vi "AutomatedTestTemplate.vi"() -> ()   [LabVIEW 2014]
uses:
  Utilities/ControlValues/ControlValues.lvclass
  Controls/Config.ctl
  Utilities/DataShare/DataShare.lvclass
  <vilib>/Utility/error.llb/DialogType.ctl
  Controls/Data.ctl
panel:
  in  "SelectPanel":i32(listbox)=-1
  out "Data":string[][](table)
  out "Status":string
  # "Blank area for constantly available displays"
  # "Blank area for constantly available displays, delete splitter if not needed"
  # "Blank area for constantly available displays"
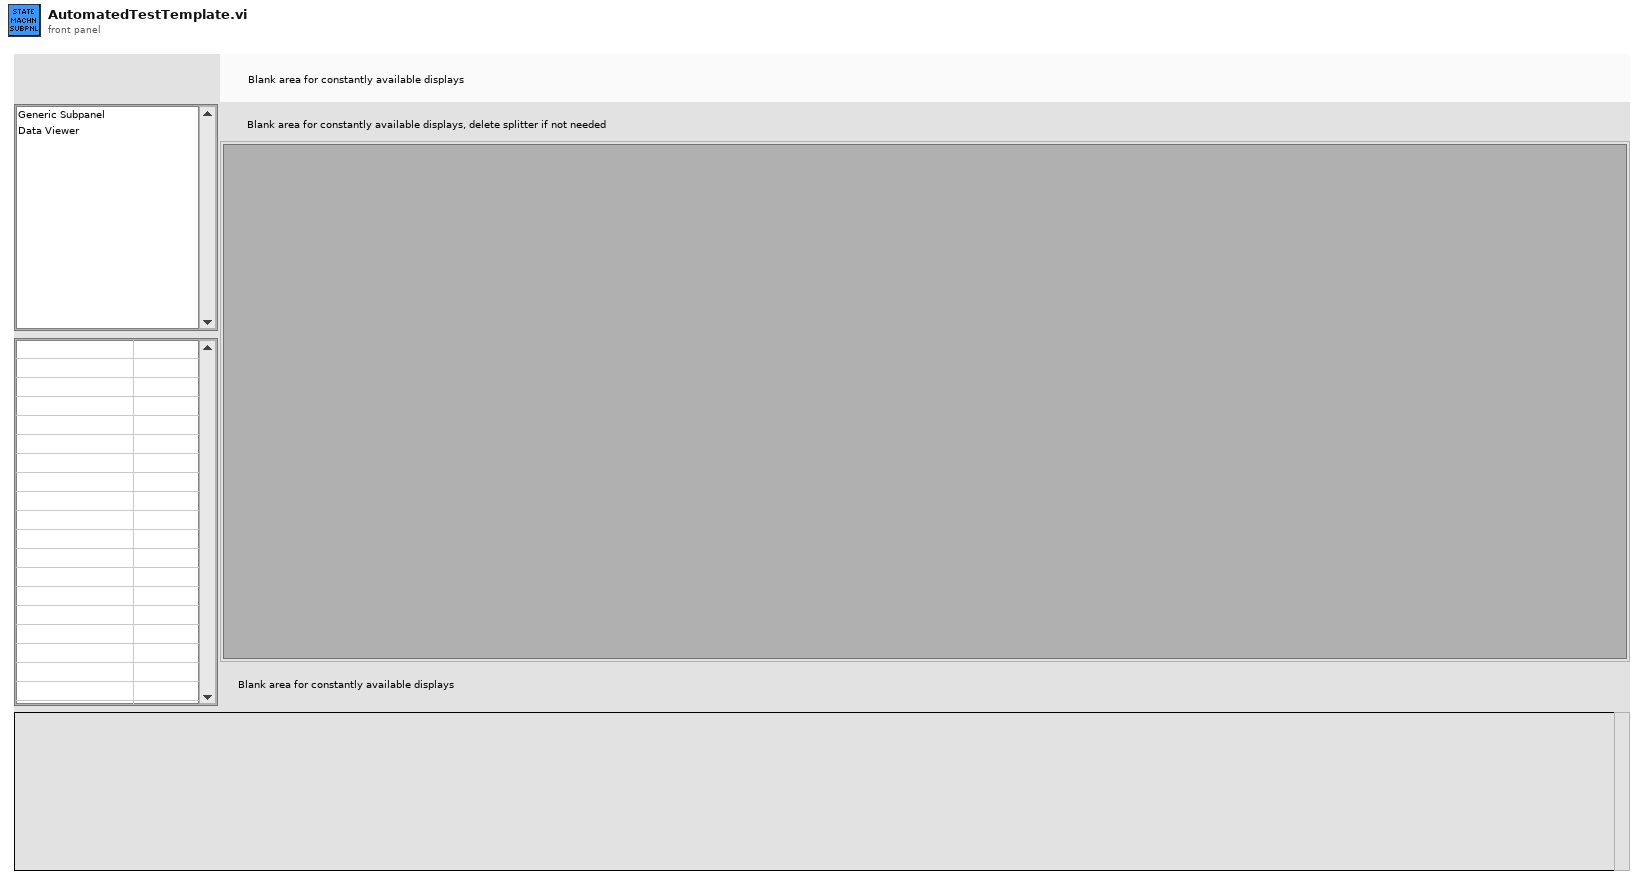
[diagram p1: front panel]
types:
  T1 = typedef "Config.ctl" = cluster{"Subpanels":cluster{"Name":string, "Pathname":string, "Type":string}[]}
  T2 = cluster{"Error":errorcluster, "SubpanelRefs":refnum<vi>[], "SubpanelRef":refnum<vi>, "ControlValues":refnum<class "ControlValues.lvclass">, "AppKind":enum32{"invalid app kind", "Development System", "Run Time System", "Student Edition", "Embedded LabVIEW", "Evaluation", "Custom"}, "LogFolder":path, "ConfigFolder":path, "Config":T1, "Hidden":T1, "Visible":T1, "Example":refnum<class "DataShare.lvclass">}
  T3 = typedef "Data.ctl" = cluster{"Names":string[], "Values":dbl[]}
  T4 = enum32{"invalid app kind", "Development System", "Run Time System", "Student Edition", "Embedded LabVIEW", "Evaluation", "Custom"}
  T5 = cluster{"Name":string, "Pathname":string, "Type":string}[]
  T6 = typedef "DialogType.ctl" = u16
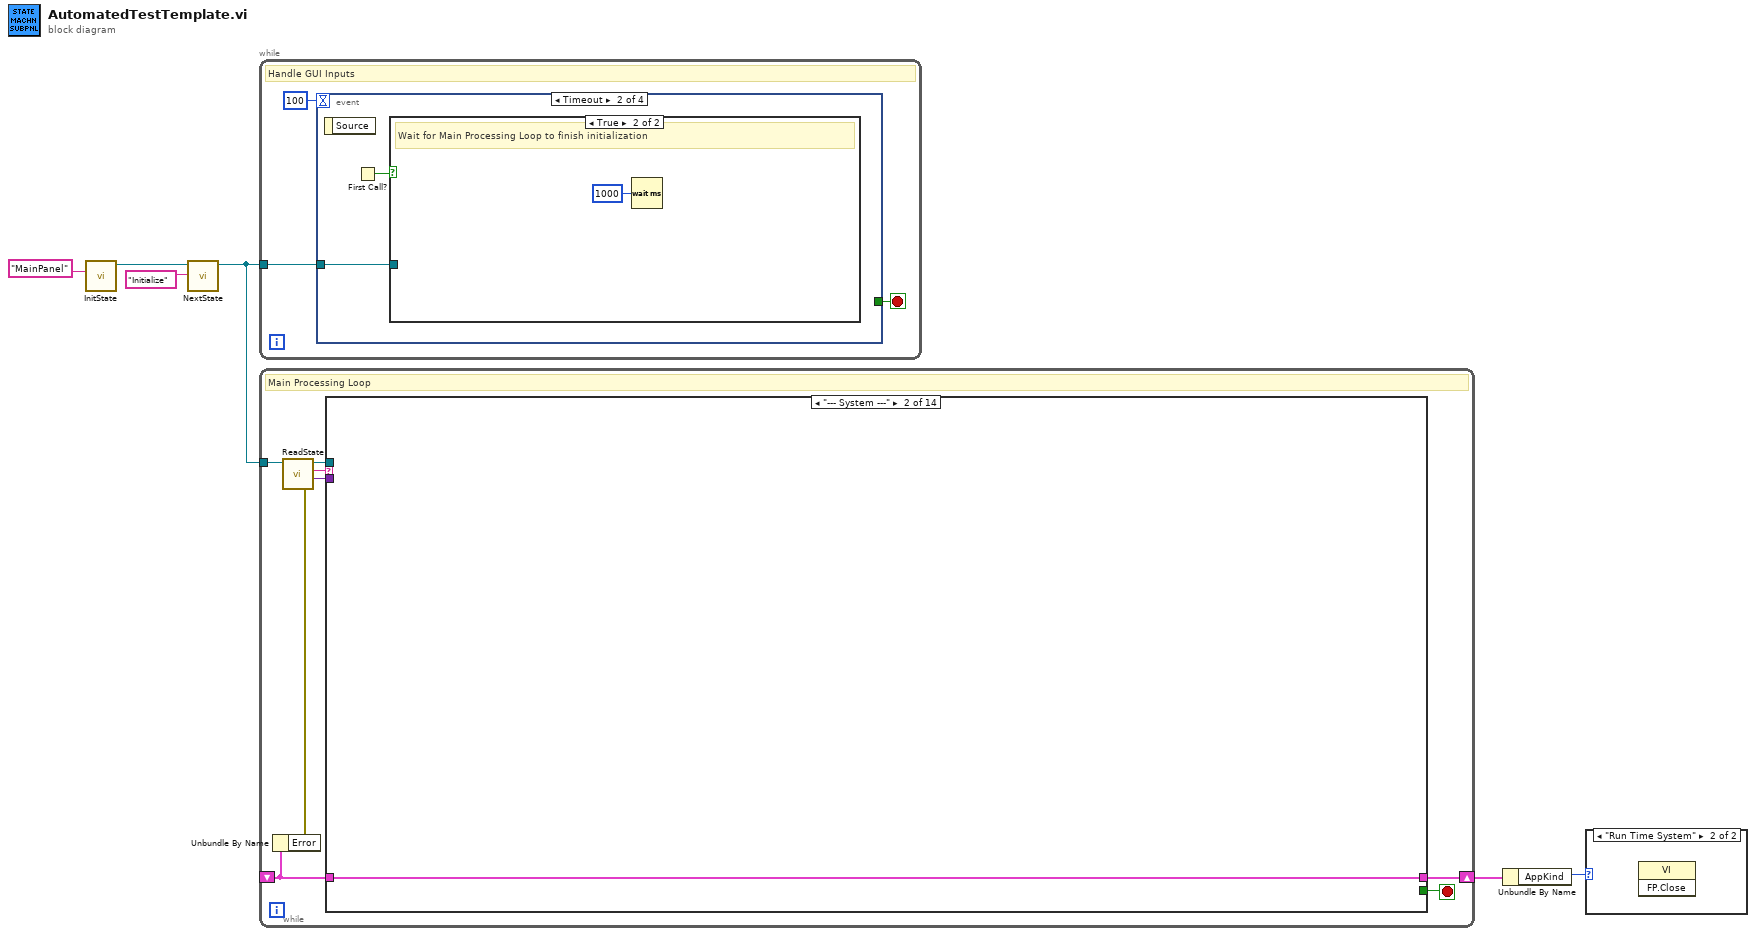
[diagram p0: block diagram]
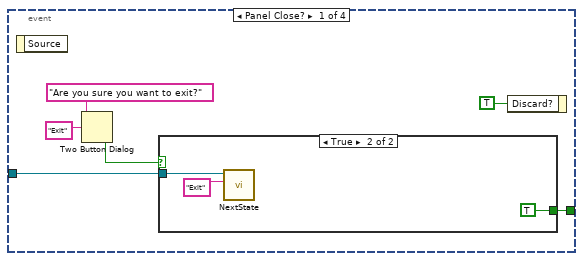
[diagram p3: hidden frame]
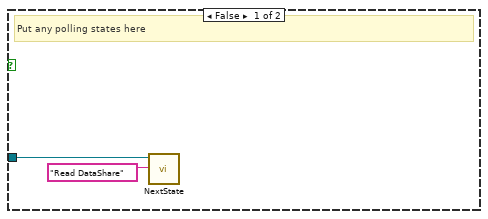
[diagram p5: hidden frame]
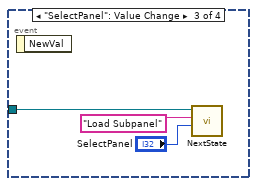
[diagram p6: hidden frame]
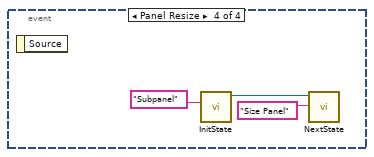
[diagram p7: hidden frame]
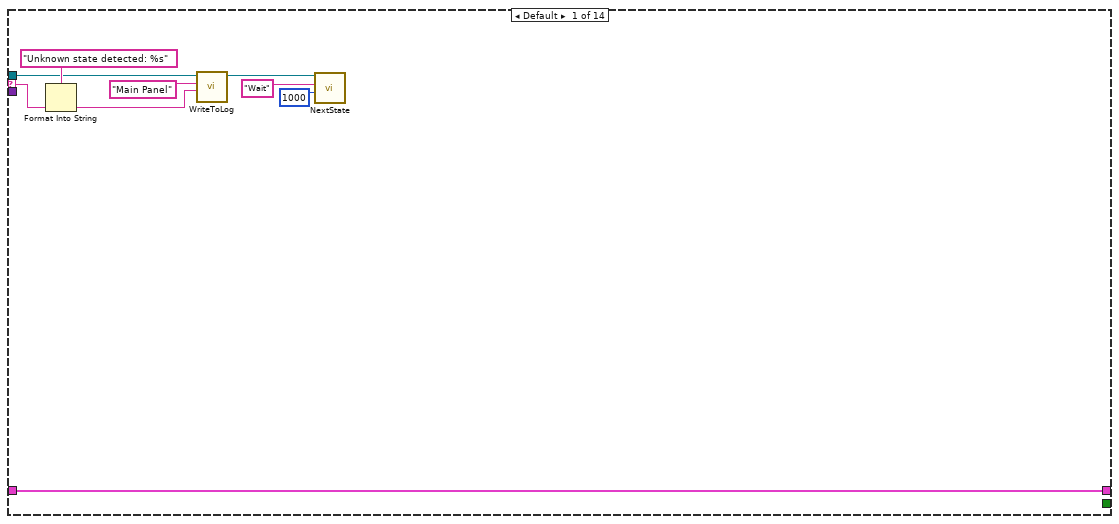
[diagram p8: hidden frame]
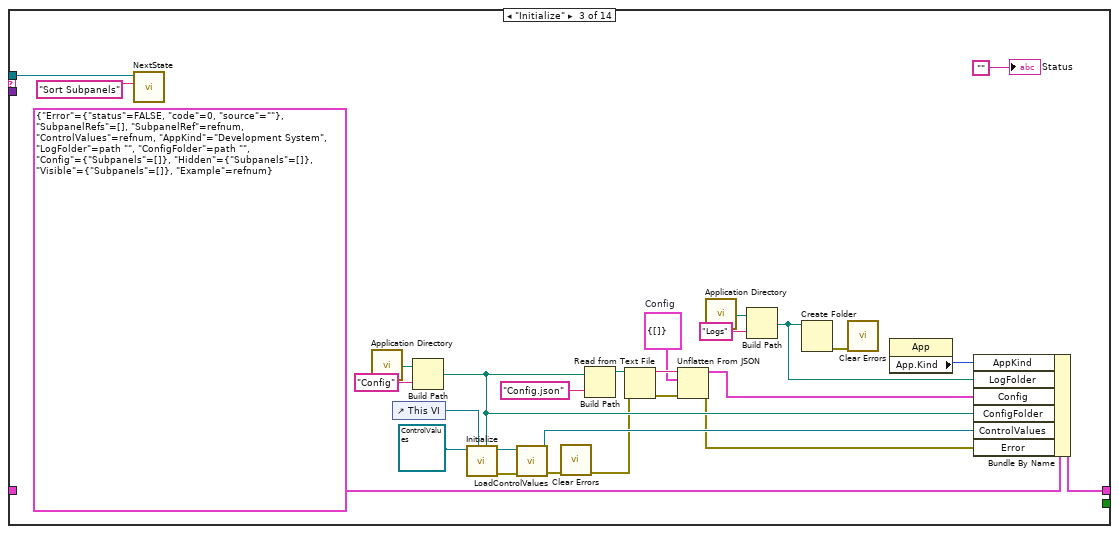
[diagram p9: hidden frame]
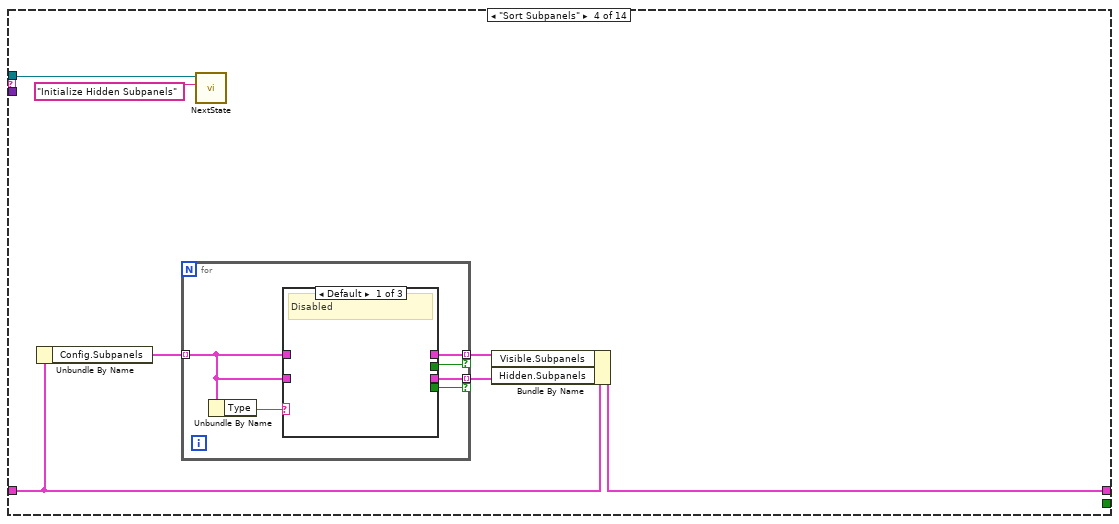
[diagram p10: hidden frame]
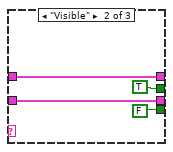
[diagram p11: hidden frame]
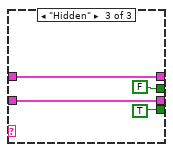
[diagram p12: hidden frame]
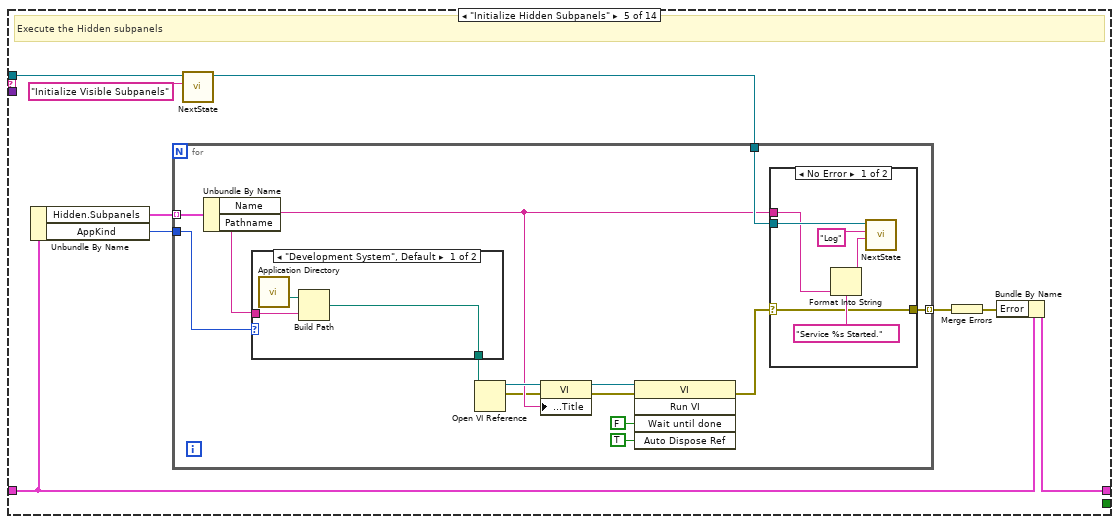
[diagram p13: hidden frame]
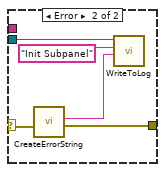
[diagram p14: hidden frame]
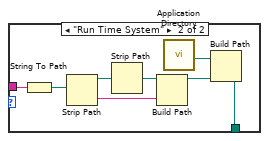
[diagram p15: hidden frame]
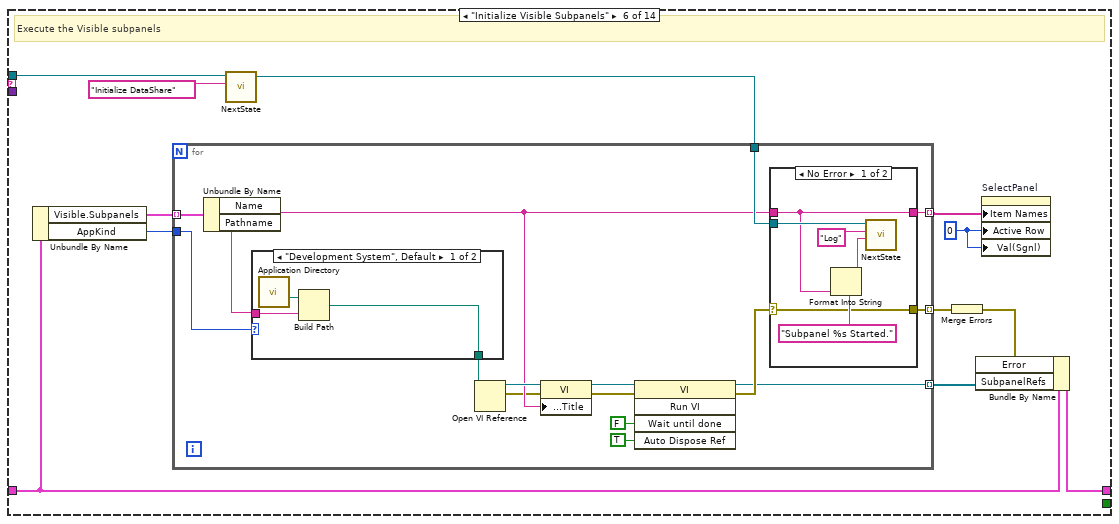
[diagram p16: hidden frame]
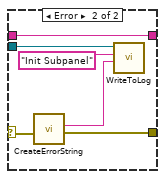
[diagram p17: hidden frame]
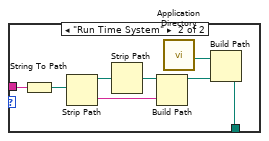
[diagram p18: hidden frame]
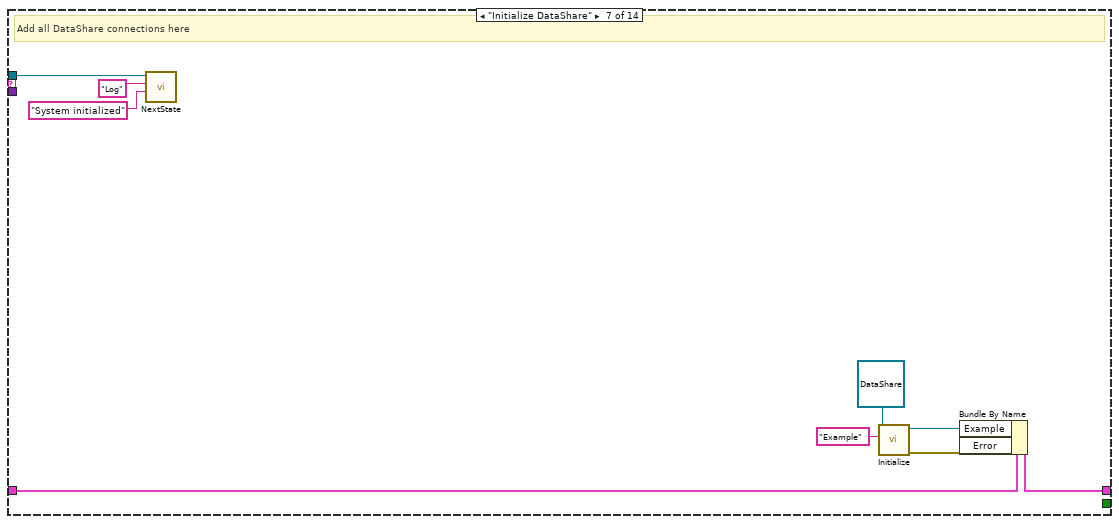
[diagram p19: hidden frame]
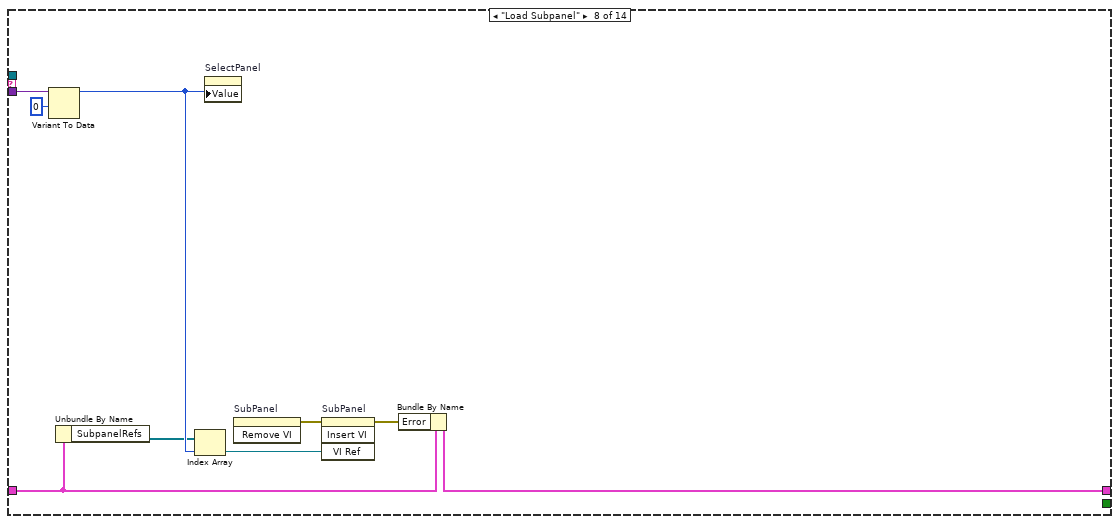
[diagram p20: hidden frame]
diagram:
  n1 = call "InitState.vi"("Name"="MainPanel" ("name (unnamed)")) -> ("Queue Out"=w2:refnum<queue>)  [unwired: 8 in, 1 out]
  n2 = call "NextState.vi"("State"="Initialize" ("element"), "Queue In"=w2) -> ("Queue Out"=w1:refnum<queue>)  [unwired: 8 in, 1 out]
  n3 = while {
    tunnel: w1 -> [w9]
    stop <- w8 stop-if-true
    # "Handle GUI Inputs"
    n4 = event shown="[1] Timeout" {
      selector: _ -> [_ _ _ _]
      dyn-events: _ -> [_ _ _ _]
      timeout: 100 -> [_ _ _ _]
      tunnel: w9 -> [w15 w19 w25 _]
      tunnel: [w10 _ _ _] -> w8
      event Panel Close? {
        n5 = event-data() -> ()  [unwired: 1 in, 1 out]
        n6 = Two Button Dialog(message="Are you sure you want to exit?", 2:"Exit" ("T button name (\"OK\")")) -> (T button?=w11:bool)  [unwired: 1 in]
        n7 = case shown="True" w11 {
          tunnel: w15 -> [_ w16]
          tunnel: [_ TRUE] -> w10
          frame False {
          }
          frame True {
            n8 = call "NextState.vi"("State"="Exit" ("element"), "Queue In"=w16) -> ()  [unwired: 8 in, 2 out]
          }
        }
        n9 = event-data("Discard?"=TRUE) -> ()  [unwired: 1 in, 1 out]
      }
      event Timeout {
        n10 = event-data() -> ()  [unwired: 1 in, 1 out]
        n11 = First Call?() -> (First Call?: T/F=w20:bool)
        n12 = case shown="True" w20 {
          tunnel: w19 -> [w22 _]
          frame False {
            # "Put any polling states here"
            n13 = call "NextState.vi"("State"="Read DataShare" ("element"), "Queue In"=w22) -> ()  [unwired: 8 in, 2 out]
          }
          frame True {
            # "Wait for Main Processing Loop to finish initialization"
            n14 = Wait (ms)(milliseconds to wait=u32 1000) -> ()  [unwired: 1 out]
          }
        }
      }
      event "SelectPanel": Value Change {
        n15 = event-data() -> ()  [unwired: 1 in, 1 out]
        n16 = call "NextState.vi"("Data"="SelectPanel", "State"="Load Subpanel", "Queue In"=w25) -> ()  [unwired: 7 in, 2 out]
      }
      event Panel Resize {
        n17 = event-data() -> ()  [unwired: 1 in, 1 out]
        n18 = call "InitState.vi"("Name"="Subpanel" ("name (unnamed)")) -> ("Queue Out"=w27:refnum<queue>)  [unwired: 8 in, 1 out]
        n19 = call "NextState.vi"("State"="Size Panel" ("element"), "Queue In"=w27) -> ()  [unwired: 8 in, 2 out]
      }
    }
  }
  n20 = while {
    tunnel: w1 -> [w35]
    shift-right: [w37] -> w6
    shift-left: _ -> [w31]
    stop <- w36 stop-if-true
    # "Main Processing Loop"
    n21 = Unbundle By Name(w31) -> ("Error"=w30:errorcluster)
    n22 = call "ReadState.vi"("Error In"=w30, "Queue In"=w35) -> ("Data"=w32:variant, "State"=w33:string, "Queue Out"=w34:refnum<queue>)  [unwired: 6 in, 1 out]
    n23 = case shown="\"--- System ---\"" w33 {
      tunnel: w34 -> [w43 _ w49 w76 w98 w142 w192 _ _ _ w258 w278 _ _]
      tunnel: w32 -> [_ _ _ _ _ _ _ w208 w224 w237 w245 _ _ _]
      selector: w33 -> [w45 _ _ _ _ _ _ _ _ _ _ _ _ _]
      tunnel: [w44 w47 w74 w77 w101 w146 w196 w206 w213 w234 w260 w277 w290 w295] -> w37
      tunnel: [_ _ _ _ _ _ _ _ _ _ _ TRUE _ _] -> w36
      tunnel: w31 -> [w44 w47 _ w80 w102 w147 w197 w205 w213 w234 w241 w277 w290 w295]
      frame Default {
        n24 = Format Into String(format string="Unknown state detected: %s", w45) -> (resulting string=w38:string)  [unwired: 2 in, 1 out]
        n25 = call "WriteToLog.vi"("Data"=w38, "Source"="Main Panel", "Queue In"=w43) -> ("Queue Out"=w42:refnum<queue>)  [unwired: 7 in, 1 out]
        n26 = call "NextState.vi"("Data"=u32 1000, "State"="Wait", "Queue In"=w42) -> ()  [unwired: 7 in, 2 out]
      }
      frame "--- System ---" {
      }
      frame "Initialize" {
        w53 = T1 {"Subpanels"=[]}  # Config
        n27 = call "NextState.vi"("State"="Sort Subpanels" ("element"), "Queue In"=w49) -> ()  [unwired: 8 in, 2 out]
        n28 = call <vilib>:"Application Directory.vi"() -> ("Application Directory"=w62:path)
        n29 = control-ref of="This VI"() -> (w69:refnum<vi>)
        n30 = Build Path(base path=w62, name or relative path="Config") -> (appended path=w57:path)
        n31 = call "Initialize.vi"("Config Path"=w57, "VI Reference"=w69, "ControlValues in"=refnum<class "ControlValues.lvclass"> refnum) -> ("error out"=w71:errorcluster, "ControlValues out"=w72:refnum<class "ControlValues.lvclass">)  [unwired: 7 in]
        n32 = call "LoadControlValues.vi"("error in"=w71, "ControlValues in"=w72) -> ("error out"=w64:errorcluster, "ControlValues out"=w70:refnum<class "ControlValues.lvclass">)  [unwired: 8 in]
        n33 = call <vilib>:"Clear Errors.vi"("error in (no error)"=w64) -> ("error out"=w54:errorcluster)  [unwired: 5 in, 1 out]
        n34 = Build Path(base path=w57, name or relative path="Config.json") -> (appended path=w58:path)
        n35 = Read from Text File(file (use dialog)=w58, error in=w54) -> (text=w59:string, error out=w60:errorcluster)  [unwired: 2 in, 2 out]
        n36 = Unflatten From JSON(JSON string=w59, type and defaults=w53, error in (no error)=w60) -> (value=w52:T1, error out=w50:errorcluster)  [unwired: 4 in]
        n37 = call <vilib>:"Application Directory.vi"() -> ("Application Directory"=w67:path)
        n38 = Build Path(base path=w67, name or relative path="Logs") -> (appended path=w56:path)
        n39 = Create Folder(path (use dialog)=w56) -> (error out=w65:errorcluster)  [unwired: 2 in, 2 out]
        n40 = call <vilib>:"Clear Errors.vi"("error in (no error)"=w65) -> ()  [unwired: 5 in, 2 out]
        n41 = property class="App"() -> ("App.Kind"=w51:T4)  [unwired: 2 in, 2 out]
        n42 = Bundle By Name(cluster=T2 {"Error"={"status"=FALSE, "code"=0, "source"=""}, "SubpanelRefs"=[], "SubpanelRef"=refnum, "ControlValues"=refnum, "AppKind"=enum."Development System", "LogFolder"=path "", "ConfigFolder"=path "", "Config"={"Subpanels"=[]}, "Hidden"={"Subpanels"=[]}, "Visible"={"Subpanels"=[]}, "Example"=refnum}, "AppKind"=w51, "LogFolder"=w56, "Config"=w52, "ConfigFolder"=w57, "ControlValues"=w70, "Error"=w50) -> (w74:T2)
        "Status" <- ""
      }
      frame "Sort Subpanels" {
        n43 = Unbundle By Name(w80) -> ("Config.Subpanels"=w81:T5)
        n44 = for {
          tunnel: w81 -> [w86] mode=indexing
          tunnel: [w85] -> w79 mode=indexing if=w82
          tunnel: [w84] -> w78 mode=indexing if=w83
          n45 = Unbundle By Name(w86) -> ("Type"=w87:string)
          n46 = case shown="Default" w87 {
            tunnel: [_ w91 w95] -> w85
            tunnel: w86 -> [_ w91 w95]
            tunnel: w86 -> [_ w90 w94]
            tunnel: [_ w90 w94] -> w84
            tunnel: [_ TRUE FALSE] -> w82
            tunnel: [_ FALSE TRUE] -> w83
            frame Default {
              # "Disabled"
            }
            frame "Visible" {
            }
            frame "Hidden" {
            }
          }
        }
        n47 = call "NextState.vi"("State"="Initialize Hidden Subpanels" ("element"), "Queue In"=w76) -> ()  [unwired: 8 in, 2 out]
        n48 = Bundle By Name(cluster=w80, "Visible.Subpanels"=w79, "Hidden.Subpanels"=w78) -> (w77:T2)
      }
      frame "Initialize Hidden Subpanels" {
        # "Execute the Hidden subpanels"
        n49 = Unbundle By Name(w102) -> ("Hidden.Subpanels"=w104:T5, "AppKind"=w103:T4)
        n50 = call "NextState.vi"("State"="Initialize Visible Subpanels", "Queue In"=w98) -> ("Queue Out"=w97:refnum<queue>)  [unwired: 8 in, 1 out]
        n51 = for {
          tunnel: w104 -> [w118] mode=indexing
          tunnel: w103 -> [w116]
          tunnel: w97 -> [w115]
          tunnel: [w105] -> w100 mode=indexing
          n52 = Unbundle By Name(w118) -> ("Name"=w109:string, "Pathname"=w117:string)
          n53 = case shown="\"Development System\", Default" w116 {
            tunnel: w117 -> [w131 w140]
            tunnel: [w130 w134] -> w114
            frame "Development System", Default {
              n54 = call <vilib>:"Application Directory.vi"() -> ("Application Directory"=w132:path)
              n55 = Build Path(base path=w132, name or relative path=w131) -> (appended path=w130:path)
            }
            frame "Run Time System" {
              n56 = String To Path(string=w140) -> (path=w139:path)
              n57 = Strip Path(path=w139) -> (stripped path=w138:path, name=w137:string)
              n58 = Strip Path(path=w138) -> (stripped path=w136:path)  [unwired: 1 out]
              n59 = Build Path(base path=w136, name or relative path=w137) -> (appended path=w135:path)
              n60 = call <vilib>:"Application Directory.vi"() -> ("Application Directory"=w133:path)
              n61 = Build Path(base path=w133, name or relative path=w135) -> (appended path=w134:path)
            }
          }
          n62 = Open VI Reference(vi path=w114) -> (vi reference=w110:refnum<vi>, error out=w106:errorcluster)  [unwired: 5 in]
          n63 = property class="VI"(reference=w110, error in=w106, "Front Panel.Title"=w109) -> (reference out=w108:refnum<vi>, error out=w107:errorcluster)
          n64 = invoke class="VI" method="Run VI"(reference=w108, error in=w107, "Wait until done"=FALSE ("Wait Until Done"), "Auto Dispose Ref"=TRUE ("Auto Dispose Reference")) -> (error out=w111:errorcluster)  [unwired: 1 in, 4 out]
          n65 = case shown="No Error" w111 {
            selector: w111 -> [w119 w129]
            tunnel: w115 -> [w123 w128]
            tunnel: w109 -> [w120 _]
            tunnel: [w119 w125] -> w105
            frame No Error {
              n66 = Format Into String(format string="Service %s Started.", w120) -> (resulting string=w121:string)  [unwired: 2 in, 1 out]
              n67 = call "NextState.vi"("Data"=w121, "State"="Log" ("element"), "Queue In"=w123) -> ()  [unwired: 7 in, 2 out]
            }
            frame Error {
              n68 = call "CreateErrorString.vi"("Error In"=w129) -> ("Error Out"=w125:errorcluster, "Error String"=w126:string)  [unwired: 9 in]
              n69 = call "WriteToLog.vi"("Data"=w126, "Source"="Init Subpanel", "Queue In"=w128) -> ()  [unwired: 7 in, 2 out]
            }
          }
        }
        n70 = Merge Errors(w100) -> (w99:errorcluster)
        n71 = Bundle By Name(cluster=w102, "Error"=w99) -> (w101:T2)
      }
      frame "Initialize Visible Subpanels" {
        w150 = 0 ("Active Row:Active Row Number")
        # "Execute the Visible subpanels"
        n72 = Unbundle By Name(w147) -> ("Visible.Subpanels"=w152:T5, "AppKind"=w151:T4)
        n73 = call "NextState.vi"("State"="Initialize DataShare" ("element"), "Queue In"=w142) -> ("Queue Out"=w141:refnum<queue>)  [unwired: 8 in, 1 out]
        n74 = for {
          tunnel: w152 -> [w168] mode=indexing
          tunnel: w151 -> [w166]
          tunnel: w141 -> [w165]
          tunnel: [w160] -> w149 mode=indexing
          tunnel: [w159] -> w148 mode=indexing
          tunnel: [w153] -> w145 mode=indexing
          n75 = Unbundle By Name(w168) -> ("Name"=w157:string, "Pathname"=w167:string)
          n76 = case shown="\"Development System\", Default" w166 {
            tunnel: w167 -> [w182 w191]
            tunnel: [w181 w185] -> w164
            frame "Development System", Default {
              n77 = call <vilib>:"Application Directory.vi"() -> ("Application Directory"=w183:path)
              n78 = Build Path(base path=w183, name or relative path=w182) -> (appended path=w181:path)
            }
            frame "Run Time System" {
              n79 = String To Path(string=w191) -> (path=w190:path)
              n80 = Strip Path(path=w190) -> (stripped path=w189:path, name=w188:string)
              n81 = Strip Path(path=w189) -> (stripped path=w187:path)  [unwired: 1 out]
              n82 = Build Path(base path=w187, name or relative path=w188) -> (appended path=w186:path)
              n83 = call <vilib>:"Application Directory.vi"() -> ("Application Directory"=w184:path)
              n84 = Build Path(base path=w184, name or relative path=w186) -> (appended path=w185:path)
            }
          }
          n85 = Open VI Reference(vi path=w164) -> (vi reference=w158:refnum<vi>, error out=w154:errorcluster)  [unwired: 5 in]
          n86 = property class="VI"(reference=w158, error in=w154, "Front Panel.Title"=w157) -> (reference out=w156:refnum<vi>, error out=w155:errorcluster)
          n87 = invoke class="VI" method="Run VI"(reference=w156, error in=w155, "Wait until done"=FALSE ("Wait Until Done"), "Auto Dispose Ref"=TRUE ("Auto Dispose Reference")) -> (reference out=w159:refnum<vi>, error out=w161:errorcluster)  [unwired: 1 in, 3 out]
          n88 = case shown="No Error" w161 {
            selector: w161 -> [w169 w179]
            tunnel: w165 -> [w173 w178]
            tunnel: w157 -> [w170 w180]
            tunnel: [w170 w180] -> w160
            tunnel: [w169 w175] -> w153
            frame No Error {
              n89 = Format Into String(format string="Subpanel %s Started.", w170) -> (resulting string=w171:string)  [unwired: 2 in, 1 out]
              n90 = call "NextState.vi"("Data"=w171, "State"="Log" ("element"), "Queue In"=w173) -> ()  [unwired: 7 in, 2 out]
            }
            frame Error {
              n91 = call "CreateErrorString.vi"("Error In"=w179) -> ("Error Out"=w175:errorcluster, "Error String"=w176:string)  [unwired: 9 in]
              n92 = call "WriteToLog.vi"("Data"=w176, "Source"="Init Subpanel", "Queue In"=w178) -> ()  [unwired: 7 in, 2 out]
            }
          }
        }
        n93 = Merge Errors(w145) -> (w144:errorcluster)
        n94 = Bundle By Name(cluster=w147, "Error"=w144, "SubpanelRefs"=w148) -> (w146:T2)
        n95 = property on="SelectPanel" class="LstBox (strict)"("Item Names"=w149, "Active Row"=w150, "Val(Sgnl)"=w150) -> ()  [unwired: 2 in, 2 out]
      }
      frame "Initialize DataShare" {
        # "Add all DataShare connections here"
        n96 = call "NextState.vi"("Data"="System initialized" ("State"), "State"="Log", "Queue In"=w192) -> ()  [unwired: 7 in, 2 out]
        n97 = call "Initialize.vi"("Name"="Example", "DataShare in"=refnum<class "DataShare.lvclass"> refnum ("DataShare.lvclass")) -> ("error out"=w195:errorcluster, "DataShare out"=w198:refnum<class "DataShare.lvclass">)  [unwired: 8 in]
        n98 = Bundle By Name(cluster=w197, "Example"=w198, "Error"=w195) -> (w196:T2)
      }
      frame "Load Subpanel" {
        n99 = Variant To Data(type=0, Variant=w208) -> (data=w203:i32)  [unwired: 1 in, 1 out]
        n100 = Unbundle By Name(w205) -> ("SubpanelRefs"=w202:refnum<vi>[])
        n101 = Index Array(array=w202, index=w203) -> (element=w201:refnum<vi>)
        n102 = property on="SelectPanel" class="LstBox (strict)"("Value"=w203) -> ()  [unwired: 2 in, 2 out]
        n103 = invoke on="SubPanel" class="SubPnl" method="Remove VI"() -> (error out=w207:errorcluster)  [unwired: 3 in, 2 out]
        n104 = invoke on="SubPanel" class="SubPnl" method="Insert VI"(error in=w207, "VI Ref"=w201) -> (error out=w204:errorcluster)  [unwired: 2 in, 3 out]
        n105 = Bundle By Name(cluster=w205, "Error"=w204) -> (w206:T2)
      }
      frame "Log", "Status" {
        n106 = Variant To Data(type="", Variant=w224) -> (data=w218:string)  [unwired: 1 in, 1 out]
        n107 = Format Date/Time String(time format string (%c)="[%m/%d/%y %H:%M:%S] ") -> (date/time string=w219:string)  [unwired: 2 in]
        n108 = feedback #1("") -> (w211:string)
        n109 = Concatenate Strings(w211, w219, w218, "\r\n") -> (w215:string)
        n110 = Unbundle By Name(w213) -> ("LogFolder"=w212:path)
        n111 = String Length(string=w215) -> (length=w216:i32)
        n112 = case shown="500000.." w216 {
          tunnel: [w225 w233] -> w214
          tunnel: w215 -> [w232 w233]
          tunnel: w212 -> [w228 _]
          tunnel: [w225 w233] -> w210
          frame 500000.. {
            n113 = Format Date/Time String(time format string (%c)="%m%d%y%H%M%S.txt" ("name or relative path")) -> (date/time string=w229:string)  [unwired: 2 in]
            n114 = Search/Split String(string=w232, offset (0)=250000) -> (substring before match=w230:string, match + rest of string=w225:string)  [unwired: 1 in, 1 out]
            n115 = Build Path(base path=w228, name or relative path=w229) -> (appended path=w227:path)
            n116 = Write to Text File(file (use dialog)=w227, text=w230) -> ()  [unwired: 2 in, 3 out]
          }
          frame Default {
          }
        }
        n117 = feedback-in #1(w210) -> ()
        n118 = property on="Status" class="Str"("Value"=w214, "Text.Scroll Position"=u32 4294967295) -> ()  [unwired: 2 in, 2 out]
      }
      frame "Wait" {
        n119 = Variant To Data(type=u32 0, Variant=w237) -> (data=w235:u32)  [unwired: 1 in, 1 out]
        n120 = Wait (ms)(milliseconds to wait=w235) -> ()  [unwired: 1 out]
      }
      frame "Error" {
        w252 = T6 0 items=["no dialog", "OK message", "continue or stop message", "OK message + warnings", "continue/stop + warnings"] ("type of dialog (OK msg:1)")
        n121 = Unbundle By Name(w241) -> ("Error"=w240:errorcluster)
        n122 = Variant To Data(type=errorcluster {"status"=FALSE, "code"=0, "source"=""} ("Error"), Variant=w245) -> (data=w242:errorcluster, error out=w243:errorcluster)  [unwired: 1 in]
        n123 = Select(t=w240, s=w243, f=w242) -> (s? t:f=w239:errorcluster)
        n124 = call <vilib>:"General Error Handler.vi"("search ni.com link visible?(T)"=FALSE, "type of dialog (OK msg:1)"=w252, "error in (no error)"=w239) -> ("source out"=w238:string, "message"=w249:string, "error out"=w253:errorcluster)  [unwired: 8 in, 2 out]
        n125 = call <vilib>:"Clear Errors.vi"("error in (no error)"=w253) -> ("error out"=w259:errorcluster)  [unwired: 5 in, 1 out]
        n126 = call "FlushState.vi"("Queue In"=w258) -> ("Queue Out"=w257:refnum<queue>)  [unwired: 9 in, 1 out]
        n127 = Search and Replace String(replace all?=TRUE ("replace all? (F)"), input string=w249, search string="\r\n", replace string=" " ("replace string (\"\")")) -> (result string=w250:string)  [unwired: 4 in, 3 out]
        n128 = Bundle By Name(cluster=w241, "Error"=w259) -> (w260:T2)
        n129 = Format Into String(format string="[%s] %s", w238, w250) -> (resulting string=w254:string)  [unwired: 2 in, 1 out]
        n130 = call "NextState.vi"("Data"=w254, "State"="Log" ("element"), "Queue In"=w257) -> ()  [unwired: 7 in, 2 out]
      }
      frame "Exit" {
        n131 = Unbundle By Name(w277) -> ("Visible.Subpanels"=w263:T5, "Hidden.Subpanels"=w262:T5, "ControlValues"=w276:refnum<class "ControlValues.lvclass">, "LogFolder"=w268:path)
        n132 = call "CloseState.vi"("Queue In"=w278) -> ()  [unwired: 10 in, 1 out]
        n133 = Build Array (concatenate)(w263, w262) -> (w261:T5)
        n134 = invoke on="SubPanel" class="SubPnl" method="Remove VI"() -> (error out=w266:errorcluster)  [unwired: 3 in, 2 out]
        n135 = for {
          tunnel: w266 -> [w284]
          tunnel: w261 -> [w283] mode=indexing
          tunnel: [w280] -> w265
          n136 = Unbundle By Name(w283) -> ("Name"=w282:string)
          n137 = call "InitState.vi"("Error In"=w284, "Name"=w282) -> ("Error Out"=w281:errorcluster, "Queue Out"=w285:refnum<queue>)  [unwired: 7 in]
          n138 = call "PriorityState.vi"("Error In"=w281, "State"="Exit", "Queue In"=w285) -> ("Error Out"=w280:errorcluster)  [unwired: 7 in, 1 out]
        }
        n139 = Format Date/Time String(time format string (%c)="%m%d%y%H%M%S.txt" ("name or relative path")) -> (date/time string=w272:string)  [unwired: 2 in]
        n140 = Build Path(base path=w268, name or relative path=w272) -> (appended path=w275:path)
        n141 = local read "Status"() -> (w274:string)
        n142 = Write to Text File(file (use dialog)=w275, text=w274) -> (error out=w271:errorcluster)  [unwired: 2 in, 2 out]
        n143 = call <vilib>:"Clear Errors.vi"("error in (no error)"=w271) -> ("error out"=w269:errorcluster)  [unwired: 5 in, 1 out]
        n144 = call "Time Delay"("error in (no error)"=w265, "Delay Time (s)"=2.0) -> ()  [unwired: 9 in, 1 out]
        n145 = disable-structure shown="Enabled" {
          disable-tunnel: [w287 w289] -> w270
          disable-tunnel: w269 -> [w287 w289]
          frame Disabled {
          }
          frame Enabled {
            n146 = local write "Status"("") -> ()
          }
        }
        n147 = call "SaveControlValues.vi"("error in"=w270, "ControlValues in"=w276) -> ("error out"=w267:errorcluster)  [unwired: 7 in, 2 out]
        n148 = call <vilib>:"Clear Errors.vi"("error in (no error)"=w267) -> ()  [unwired: 5 in, 2 out]
      }
      frame "--- DataShare ---" {
      }
      frame "Read DataShare" {
        # "Create a custom DataShare state for each connection"
        n149 = Unbundle By Name(w295) -> ("Example"=w294:refnum<class "DataShare.lvclass">)
        n150 = call "Read.vi"("Timeout"=0, "DataShare in"=w294) -> ("Timed Out?"=w293:bool, "Data"=w292:variant)  [unwired: 6 in, 2 out]
        n151 = case shown="False" w293 {
          tunnel: w292 -> [w303 _]
          frame False {
            # "Replace this with required data type"
            n152 = Variant To Data(type=T3 {"Names"=[], "Values"=[]} ("Data"), Variant=w303) -> (data=w301:T3)  [unwired: 1 in, 1 out]
            n153 = Unbundle By Name(w301) -> ("Names"=w298:string[], "Values"=w300:dbl[])
            n154 = Number To Fractional String(number=w300, precision (6)=i16 3) -> (F-format string=w297:string[])  [unwired: 2 in]
            n155 = for {
              tunnel: w298 -> [w306] mode=indexing
              tunnel: w297 -> [w305] mode=indexing
              tunnel: [w304] -> w296 mode=indexing
              n156 = Build Array(w306, w305) -> (w304:string[])
            }
            "Data" <- w296
          }
          frame True {
          }
        }
      }
    }
  }
  n157 = Unbundle By Name(w6) -> ("AppKind"=w3:T4)
  n158 = case shown="\"Run Time System\"" w3 {
    frame Default {
    }
    frame "Run Time System" {
      n159 = invoke class="VI" method="FP.Close"() -> ()  [unwired: 3 in, 3 out]
    }
  }
